vi "add.vi"() -> ()   [LabVIEW 2025]
uses:
  ArrayInc/x64/Release/ArrayInc.dll
panel:
  out "element":u8
  out "1/x":dbl
  out "x = y?":bool
  out "x-y 2":dbl format="%#.11f"
  out "sum 2":u8
  out "sum":u8
  out "x-y":dbl
  # "r"
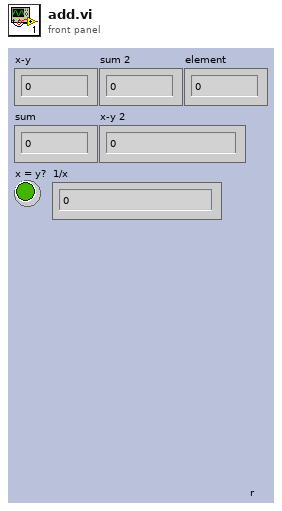
[diagram p1: front panel]
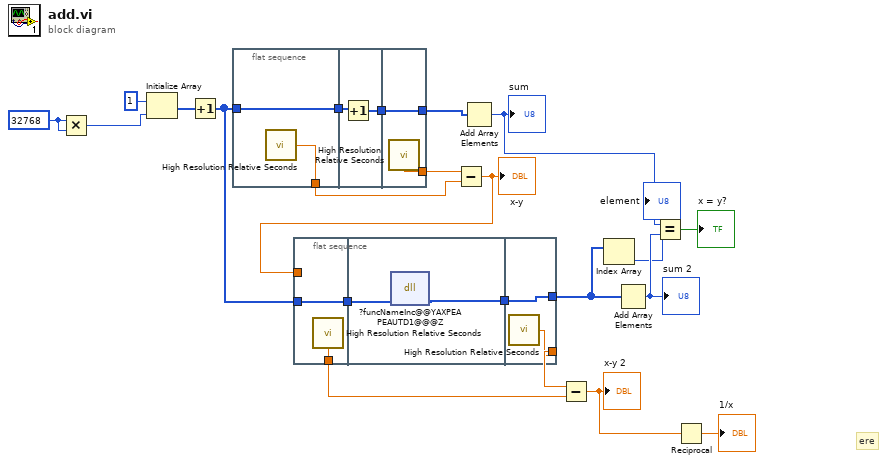
[diagram p0: block diagram]
diagram:
  w21 = 32768 ("x")
  # "ere"
  n1 = Multiply(x=w21, y=w21) -> (x*y=w20:i32)
  n2 = Initialize Array(u8 1 ("element"), w20) -> (w19:u8[])
  n3 = Increment(x=w19) -> (x+1=w13:u8[])
  n4 = flat-sequence {
    tunnel: w13 -> [w24]
    tunnel: [w24] -> w18
    tunnel: [w23] -> w15
    tunnel: w18 -> [w26]
    tunnel: [w25] -> w17
    tunnel: w17 -> [w28]
    tunnel: [w28] -> w14
    tunnel: [w27] -> w16
    frame #0 {
      n5 = call <vilib>:"High Resolution Relative Seconds.vi"() -> ("relative seconds"=w23:dbl)
    }
    frame #1 {
      n6 = Increment(x=w26) -> (x+1=w25:u8[])
    }
    frame #2 {
      n7 = call <vilib>:"High Resolution Relative Seconds.vi"() -> ("relative seconds"=w27:dbl)
    }
  }
  n8 = flat-sequence {
    tunnel: w13 -> [w30]
    tunnel: [w30] -> w12
    tunnel: [w29] -> w9
    tunnel: w8 -> [_]
    tunnel: w12 -> [w32]
    tunnel: [w31] -> w11
    tunnel: [w34] -> w2
    tunnel: w11 -> [w34]
    tunnel: [w33] -> w10
    frame #0 {
      n9 = call <vilib>:"High Resolution Relative Seconds.vi"() -> ("relative seconds"=w29:dbl)
    }
    frame #1 {
      n10 = dll-call lib="C:/Users/Andrey/Desktop/ArrayIncMSVC/ArrayInc/x64/Release/ArrayInc.dll" fn="?funcNameInc@@YAXPEAPEAUTD1@@@Z"("array"=w32) -> ("array"=w31:u8[])  [unwired: 4 in, 2 out]
    }
    frame #2 {
      n11 = call <vilib>:"High Resolution Relative Seconds.vi"() -> ("relative seconds"=w33:dbl)
    }
  }
  n12 = Subtract(x=w16, y=w15) -> (x-y=w8:dbl)
  "x-y" <- w8
  n13 = Add Array Elements(numeric array=w14) -> (sum=w6:u8)
  "sum" <- w6
  n14 = Subtract(x=w10, y=w9) -> (x-y=w4:dbl)
  "x-y 2" <- w4
  n15 = Index Array(array=w2) -> (element=→"element":u8)  [unwired: 1 in]
  n16 = Add Array Elements(numeric array=w2) -> (sum=w7:u8)
  "sum 2" <- w7
  n17 = Equal?(x=w6, y=w7) -> (x = y?=→"x = y?":bool)
  n18 = Reciprocal(x=w4) -> (1/x=→"1/x":dbl)
